vi "LuaPrintStack.vi"(0 "L":u64, 1 "Path":path) -> ()   [LabVIEW 2014]
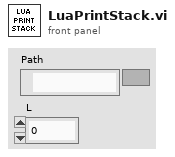
[diagram p1: front panel]
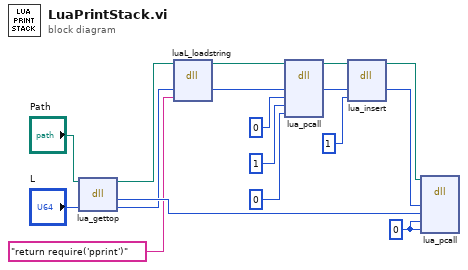
[diagram p0: block diagram]
diagram:
  w17 = 0 ("nargs")
  n1 = dll-call lib="lua5.dll" fn="lua_gettop"(path in="Path", "L"="L") -> (path out=w9:path, w11:i32, "L"=w10:u64)  [unwired: 2 in, 1 out]
  n2 = dll-call lib="lua5.dll" fn="luaL_loadstring"(path in=w9, "L"=w10, "str"="return require('pprint')") -> (path out=w6:path, "L"=w5:u64)  [unwired: 4 in, 1 out]
  n3 = dll-call lib="lua5.dll" fn="lua_pcall"(path in=w6, "L"=w5, "nargs"=0, "nresults"=1, "errfunc"=0) -> (path out=w13:path, "L"=w12:u64)  [unwired: 6 in, 1 out]
  n4 = dll-call lib="lua5.dll" fn="lua_insert"(path in=w13, "L"=w12, "idx"=1) -> (path out=w15:path, "L"=w16:u64)  [unwired: 4 in, 1 out]
  n5 = dll-call lib="lua5.dll" fn="lua_pcall"(path in=w15, "L"=w16, "nargs"=w11, "nresults"=w17, "errfunc"=w17) -> ()  [unwired: 7 in, 2 out]
